vi "Find Element and Attributes.vi"(6 "max offset":i32, 8 "offset (0)":i32, 11 "XML String In":string) -> (0 "offset past match":i32, 2 "tag with attributes":string)   [LabVIEW 2011]
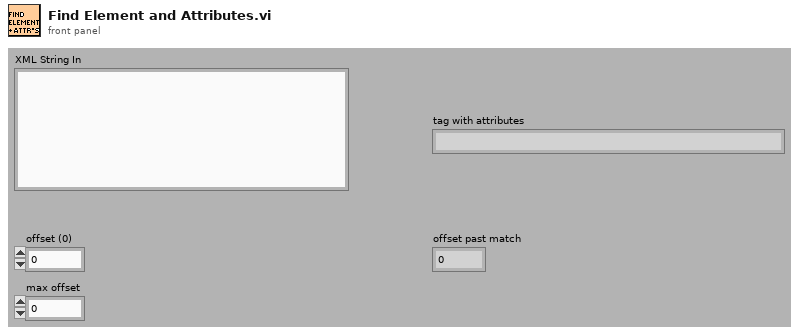
[diagram p1: front panel]
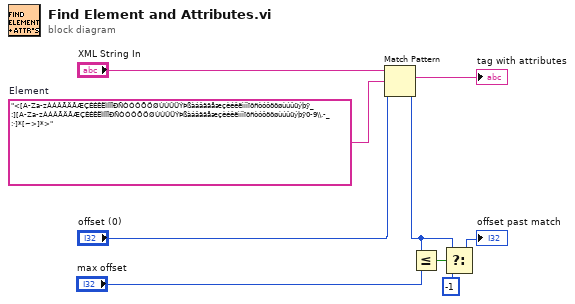
[diagram p0: block diagram]
diagram:
  w8 = "<[A-Za-zÀÁÂÃÄÅÆÇÈÉÊËÌÍÎÏÐÑÒÓÔÕÖØÙÚÛÜÝÞßàáâãäåæçèéêëìíîïðñòóôõöøùúûüýþÿ_:][A-Za-zÀÁÂÃÄÅÆÇÈÉÊËÌÍÎÏÐÑÒÓÔÕÖØÙÚÛÜÝÞßàáâãäåæçèéêëìíîïðñòóôõöøùúûüýþÿ0-9\\.-_:·]*[~>]*>"  # Element
  n1 = Match Pattern(string="XML String In", regular expression=w8, offset (0)="offset (0)") -> (match substring=→"tag with attributes":string, offset past match=w4:i32)  [unwired: 2 out]
  n2 = Less Or Equal?(x=w4, y="max offset") -> (x <= y?=w5:bool)
  n3 = Select(t=w4, s=w5, f=-1) -> (s? t:f=→"offset past match":i32)
